vi "Dwell Time.vi"(7 "Read Value? (F)":bool, 8 "error in (no error)":errorcluster, 10 "Dwell Time (1E0 s)":dbl=1.0 min=0.002 max=60.0 format="%_1e", 11 "VISA resource name":refnum<visa-resource-name>) -> (0 "error out":errorcluster, 2 "Dwell Time":dbl=1.0 format="%_1e", 3 "VISA resource name out":refnum<visa-resource-name>)   [LabVIEW 2013, in "SRS SR400.lvlib"]
doc: "<B>DT { x }</B>\n\nThe DT command reads and sets the dwell time. If x is absent, the dwell time is returned. If x is included, the dwell time is set to x seconds where 2E-3 <= x <= 6E1. If x = 0, the dwell is set to EXTERNAL. Only the most significant digit of x is used so \"DT 2E-3\" , \"DT .0022\" , \"DT 2.2E-3\" all set the dwell to 2 ms."
uses:
  <instrlib>/SRS SR400/SRS SR400.lvlib
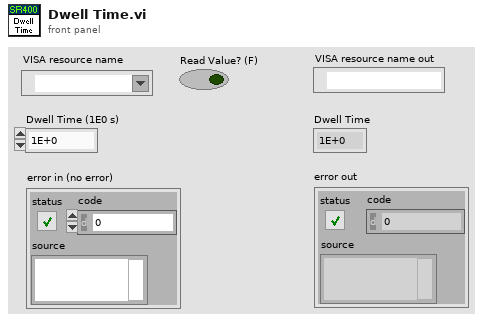
[diagram p1: front panel]
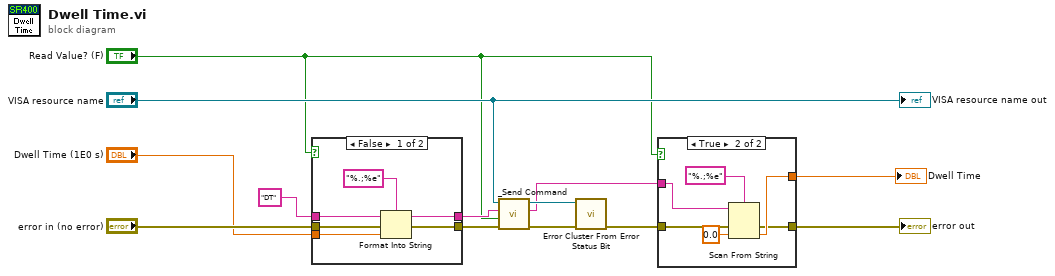
[diagram p0: block diagram]
diagram:
  n1 = case shown="False" "Read Value? (F)" {
    tunnel: "error in (no error)" -> [w19 w20]
    tunnel: "DT" ("command") -> [w17 w21]
    tunnel: [w16 w21] -> w11
    tunnel: [w15 w20] -> w10
    tunnel: "Dwell Time (1E0 s)" -> [w14 _]
    frame False {
      n2 = Format Into String(format string="%.;%e", initial string=w17, error in=w19, w14) -> (resulting string=w16:string, error out=w15:errorcluster)
    }
    frame True {
    }
  }
  n3 = call <instrlib>:"_Send Command.vi"("error in (no error)"=w10, "Read Value? (F)"="Read Value? (F)", "Command"=w11, "VISA resource name"="VISA resource name") -> ("error out"=w7:errorcluster, "Response"=w4:string, "VISA resource name out"=w8:refnum<visa-resource-name>)  [unwired: 5 out]
  n4 = call <instrlib>:"Error Cluster From Error Status Bit.vi"("error in (no error)"=w7, "VISA resource name"=w8) -> ("error out"=w5:errorcluster)  [unwired: 8 in, 1 out]
  n5 = case shown="True" "Read Value? (F)" {
    tunnel: w5 -> [w22 w28]
    tunnel: w4 -> [_ w27]
    tunnel: [_ w24] -> w3
    tunnel: [w22 w23] -> w2
    frame False {
    }
    frame True {
      n6 = Scan From String(format string="%.;%e", input string=w27, error in=w28, default 1=0.0 ("default value 1")) -> (error out=w23:errorcluster, output 1=w24:dbl)  [unwired: 1 in, 2 out]
    }
  }
  "error out" <- w2
  "Dwell Time" <- w3
  "VISA resource name out" <- "VISA resource name"
